vi "parse_joint_state.vi"(4 "error in":errorcluster, 7 "msg in":string) -> (0 "error out":errorcluster, 1 "Header":T1, 2 "ROS Joint States":T2, 3 "msg out":string)   [LabVIEW 2013]
uses:
  primitives/subs/parse_string_array.vi
  primitives/subs/parse_float64_array.vi
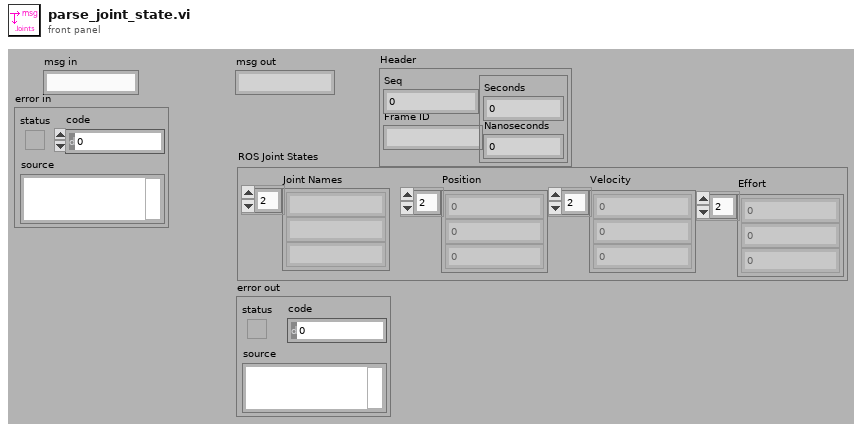
[diagram p1: front panel]
types:
  T1 = cluster{"Seq":u32, "Frame ID":string, cluster{"Seconds":i32, "Nanoseconds":i32}}
  T2 = cluster{"Joint Names":string[], "Position":dbl[], "Velocity":dbl[], "Effort":dbl[]}
  T3 = cluster{"Seq":u32, "Frame ID":string, "Timestamp":cluster{"Seconds":i32, "Nanoseconds":i32}}
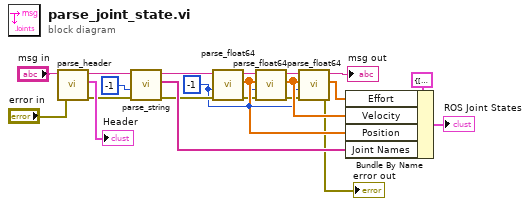
[diagram p0: block diagram]
diagram:
  w1 = -1
  n1 = call "parse_header.vi"("error in"="error in", "msg in"="msg in") -> ("error out"=w4:errorcluster, "Header"=→"Header":T3, "msg out"=w19:string)  [unwired: 3 in]
  n2 = call-poly "parse_string.vi"("error in"=w4, "Array Size"=-1, "msg in"=w19) -> ("error out"=w5:errorcluster, "strings"=w15:string[], "msg out"=w17:string)  [unwired: 2 in]
  n3 = call-poly "parse_float64.vi"("error in"=w5, "Array Size"=w1, "msg in"=w17) -> ("error out"=w7:errorcluster, "number"=w12:dbl[], "msg out"=w14:string)  [unwired: 2 in]
  n4 = call-poly "parse_float64.vi"("error in"=w7, "Array Size"=w1, "type"=w12, "msg in"=w14) -> ("error out"=w6:errorcluster, "number"=w11:dbl[], "msg out"=w13:string)  [unwired: 1 in]
  n5 = call-poly "parse_float64.vi"("error in"=w6, "Array Size"=w1, "type"=w11, "msg in"=w13) -> ("error out"=→"error out":errorcluster, "number"=w10:dbl[], "msg out"=→"msg out":string)  [unwired: 1 in]
  n6 = Bundle By Name(cluster=T2 {"Joint Names"=["head_nod", "head_pan", "left_e0", "left_e1", "left_s0", "left_s1", "left_w0", "left_w1", "left_w2", "right_e0", "right_e1", "right_s0", "right_s1", "right_w0", "right_w1", "right_w2", "torso_t0"], "Position"=[0.0, -1.625976560642051, -3.6035156208823826, 89.31884755418834, 23.00537106746253, 2.7246093718866797, 106.83105456542773, 6.679687492367345, 12.50244139196388, -1.8457031228909766, 62.55615227226917, 50.866699160626325, -28.60839840481014, -69.14794913973695, 39.814453079505356, 51.02050775420057, -719.9780265210551], "Velocity"=[0.0, 0.04291534418924332, -0.944137572163353, -1.4376640303396513, -0.3218650814193249, -0.6651878349332715, 0.34332275351394653, 1.2445449814880565, 1.0514259326364612, -1.008510588447218, 2.6822090118277075, 0.0, 0.8797645558794881, -53.92312997378423, -21.43621442252704, -0.2145767209462166, 0.0], "Effort"=[0.0, 0.0, -59.12924445750096, -26.12687545796554, -7.104676659622208, 168.67877488651436, 2.521014298575622, 20.626480624709636, -2.521014298575622, -121.23786944968221, -762.0338675239949, 8.708958485988513, -1210.7744126704558, -90.75651474872241, 29.56462222875048, -13.750987083139757, -1173.417564427926]} ("ROS Joint States"), "Effort"=w10, "Velocity"=w11, "Position"=w12, "Joint Names"=w15) -> (→"ROS Joint States":T2)
